vi "Set Transfer Line Color.vi"(8 "error in (no error)":errorcluster, 10 "Round Color Box":u32(colorbox), 11 "AMS Gas in":refnum<class "AMS Gas.lvclass">) -> (0 "error out":errorcluster, 3 "AMS Gas out":refnum<class "AMS Gas.lvclass">)   [LabVIEW 2015, in "AMS UI.lvlib" / "AMS Gas.lvclass"]
uses:
  AMS Gas.lvclass
  AMS Gas.lvclass/AMS Gas.ctl
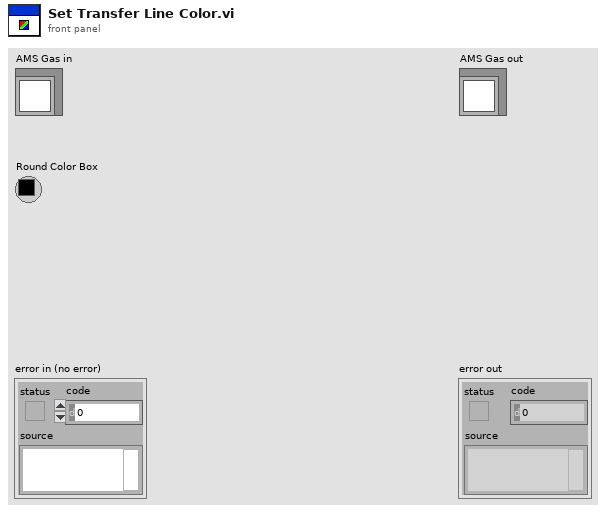
[diagram p1: front panel]
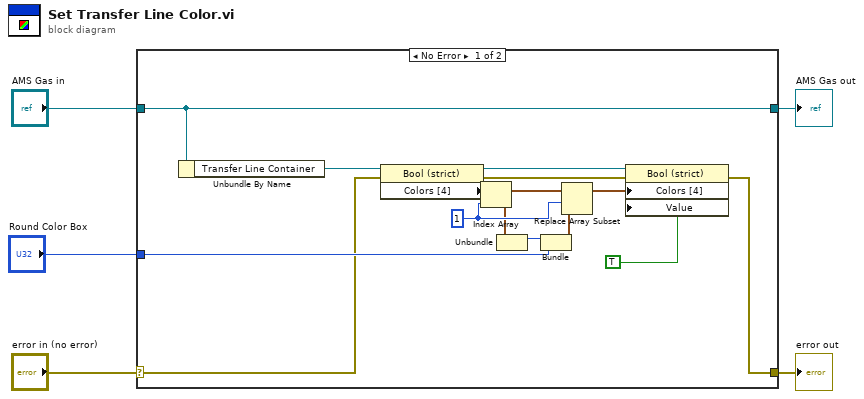
[diagram p0: block diagram]
diagram:
  n1 = case shown="No Error" "error in (no error)" {
    selector: "error in (no error)" -> [w7 w21]
    tunnel: [w6 w21] -> w4
    tunnel: [w19 w20] -> w2
    tunnel: "AMS Gas in" -> [w19 w20]
    tunnel: "Round Color Box" -> [w18 _]
    frame No Error {
      w14 = 1 ("index")
      n2 = Unbundle By Name(w19) -> ("Transfer Line Container"=w8:refnum<vi>)
      n3 = property class="Bool (strict)"(reference=w8, error in=w7) -> (reference out=w17:refnum<vi>, error out=w16:errorcluster, "Colors [4]"=w15:cluster{u32, u32}[])
      n4 = Index Array(array=w15, index=w14) -> (element=w9:cluster{u32, u32})
      n5 = Unbundle(w9) -> (w10:u32)  [unwired: 1 out]
      n6 = Bundle(w10, "Round Color Box"=w18) -> (w13:cluster{u32, "Round Color Box":u32})  [unwired: 1 in]
      n7 = Replace Array Subset(array=w15, new element=w13, index=w14) -> (w12:cluster{u32, u32}[])
      n8 = property class="Bool (strict)"(reference=w17, error in=w16, "Colors [4]"=w12, "Value"=TRUE) -> (error out=w6:errorcluster)  [unwired: 1 out]
    }
    frame Error {
    }
  }
  "error out" <- w4
  "AMS Gas out" <- w2
